vi "Move Robot.vi"(0 "Power (-100 to 100)\n0 = Stop/Brake\n-128 = Stop/Coast":i8(slide) scale=-100.0..100.0, 1 "Mode":enum16{"Constent Speed", "Rotation", "Stop"}(ring), 2 "Move mode":T1(ring), 3 "Robot Target (mm,Rotation)":i32) -> ()   [LabVIEW 2015]
panel:
  out "Busy":bool
  # "1770 = 1 Rotation"
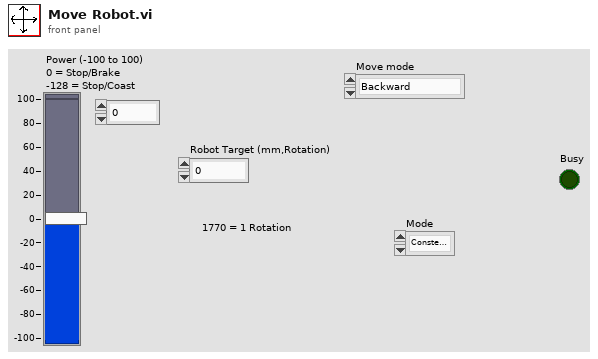
[diagram p1: front panel]
types:
  T1 = enum16{"Backward", "Forward", "Left", "Right", "Rotate Left", "Rotate Right"}
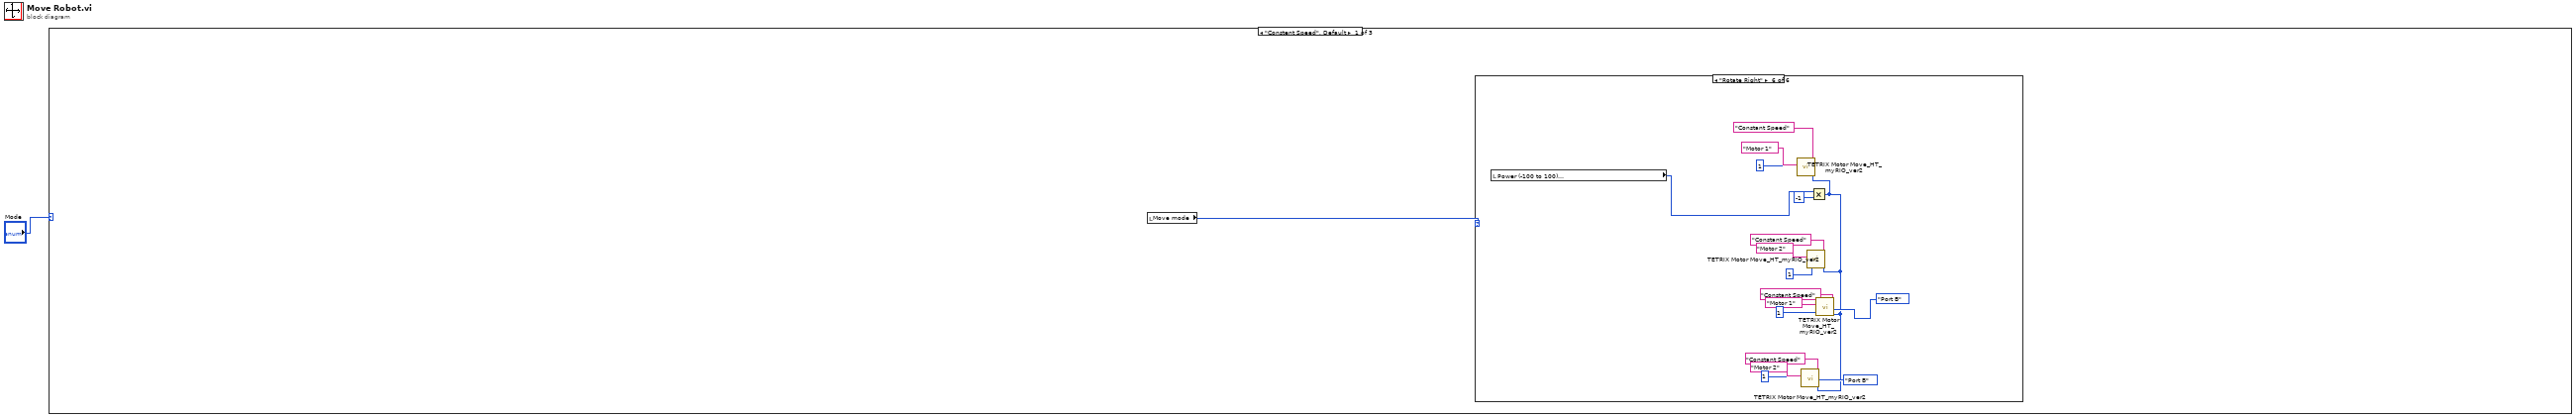
[diagram p0: block diagram]
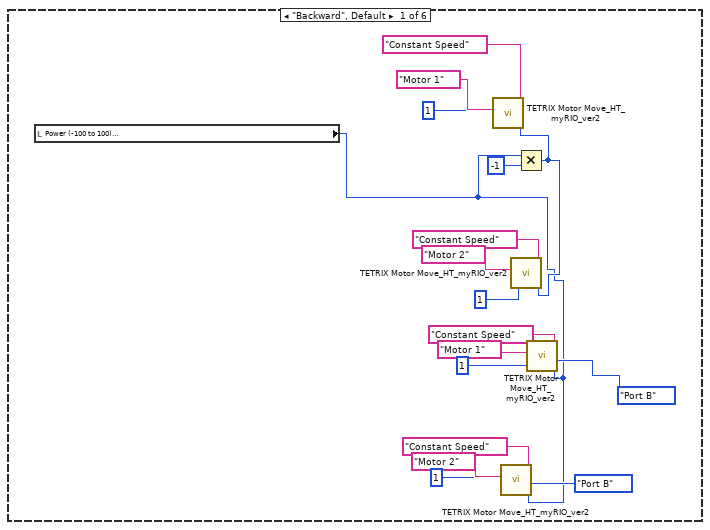
[diagram p2: hidden frame]
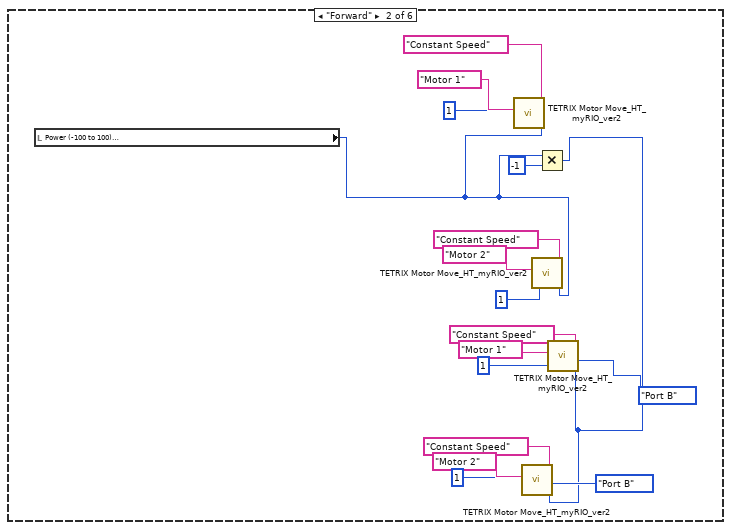
[diagram p3: hidden frame]
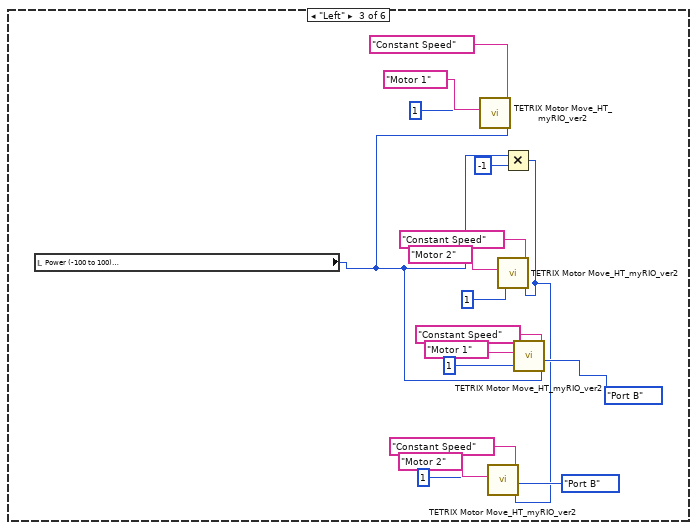
[diagram p4: hidden frame]
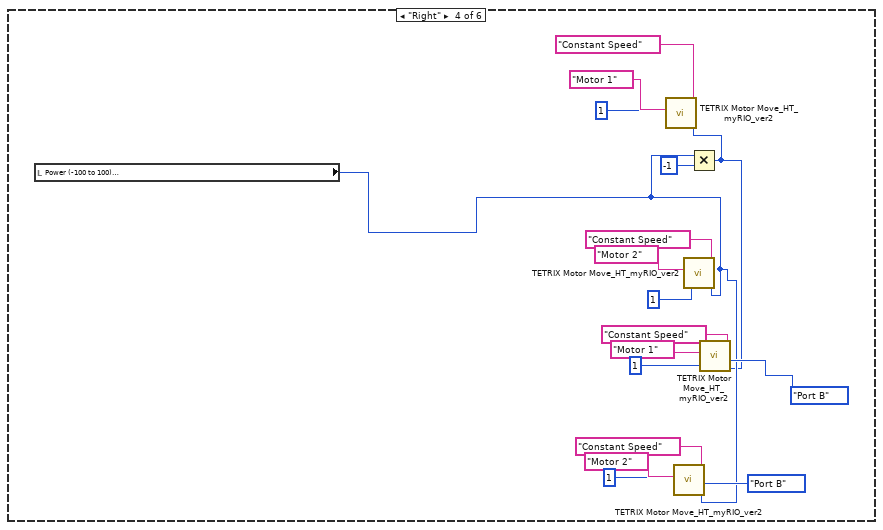
[diagram p5: hidden frame]
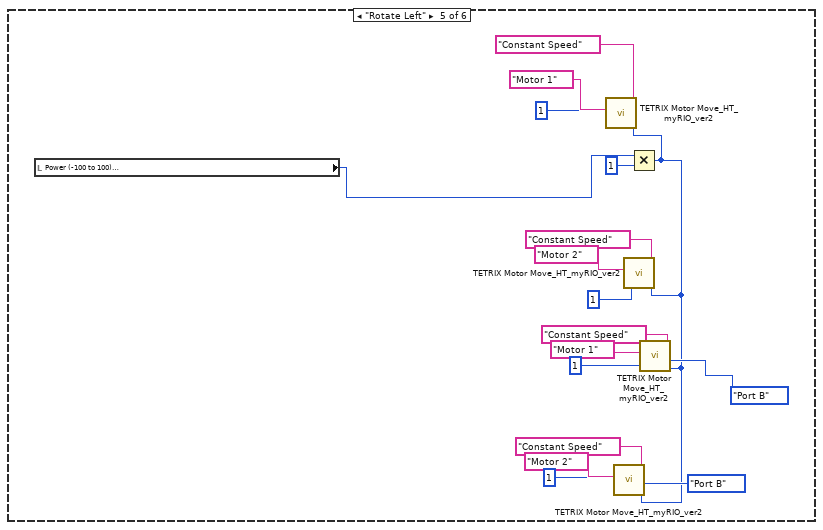
[diagram p6: hidden frame]
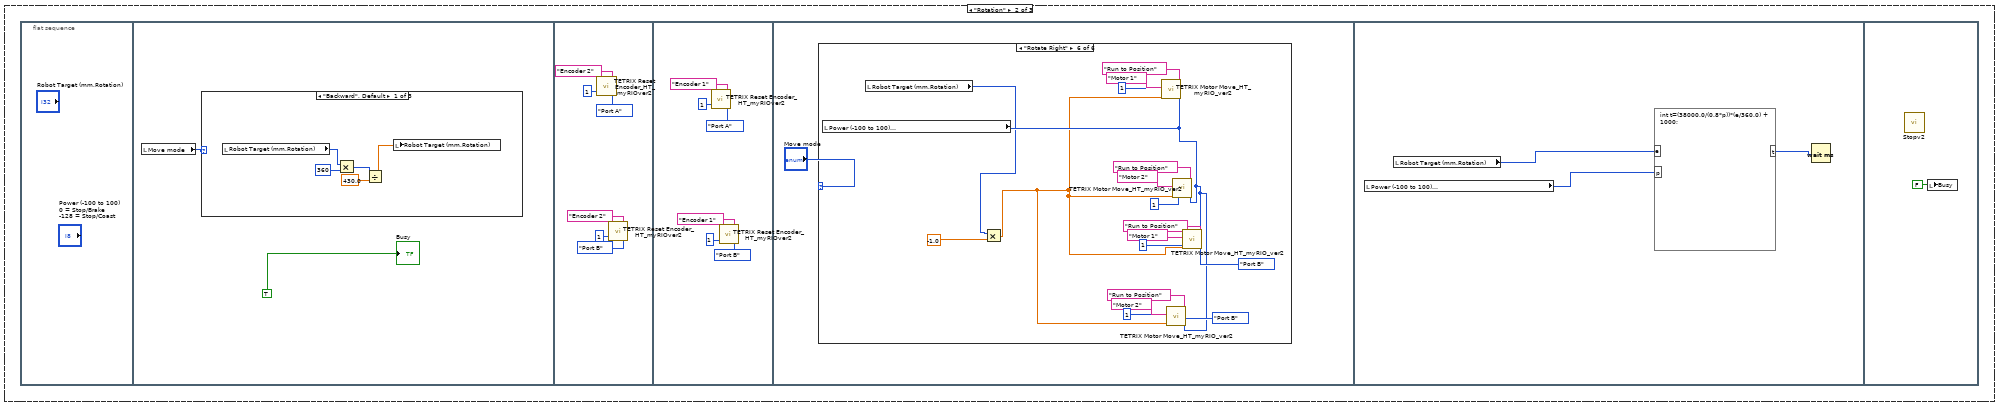
[diagram p7: hidden frame]
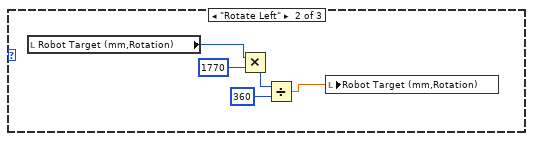
[diagram p8: hidden frame]
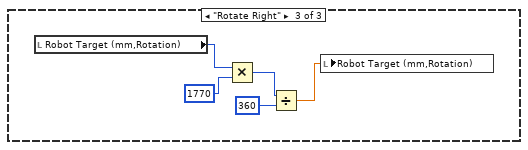
[diagram p9: hidden frame]
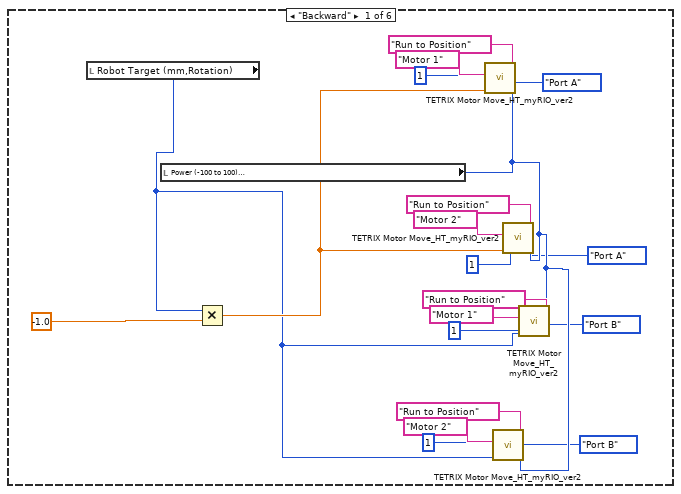
[diagram p10: hidden frame]
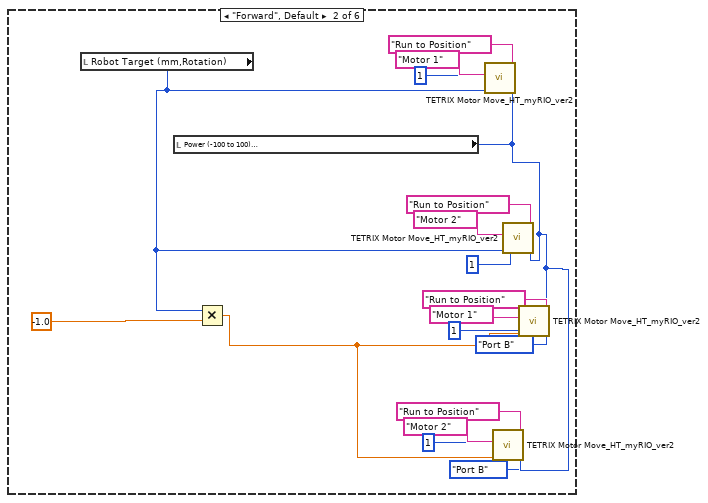
[diagram p11: hidden frame]
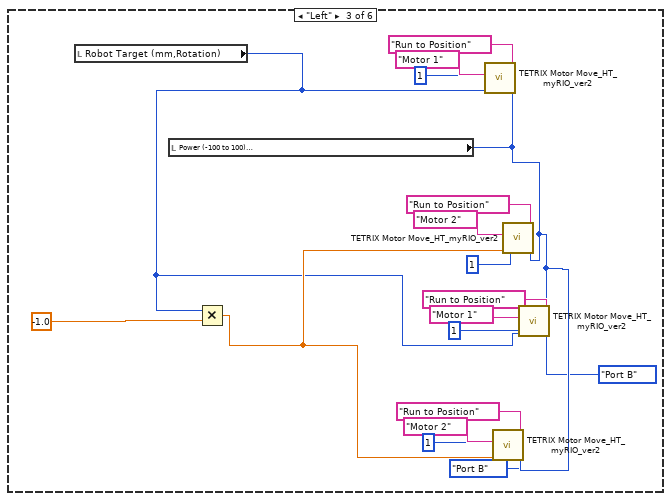
[diagram p12: hidden frame]
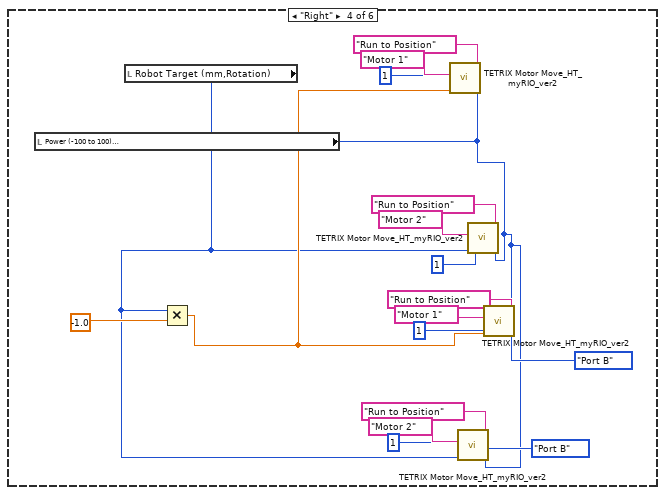
[diagram p13: hidden frame]
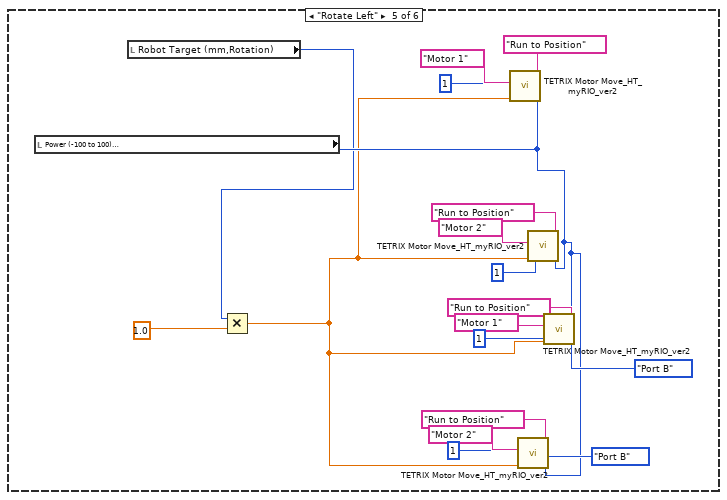
[diagram p14: hidden frame]
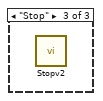
[diagram p15: hidden frame]
diagram:
  n1 = case shown="\"Constent Speed\", Default" "Mode" {
    frame "Constent Speed", Default {
      n2 = local read "Move mode"() -> (w2:T1)
      n3 = case shown="\"Rotate Right\"" w2 {
        frame "Backward", Default {
          n4 = local read "Power (-100 to 100)\n0 = Stop/Brake\n-128 = Stop/Coast"() -> (w3:i8)
          n5 = call "TETRIX Motor Move_HT_myRIO_ver2.vi"("Select Channel"="Motor 2", "Controller Daisy Chain Position: 1 - 4"=u8 1, "Control Mode"="Constant Speed", "Port"=enum16{"Port A", "Port B", ""}."Port B", "Power (-100 to 100)\n0 = Stop/Brake\n-128 = Stop/Coast"=w3) -> ()  [unwired: 3 in, 1 out]
          n6 = Multiply(x=w3, y=i8 -1) -> (x*y=w4:i8)
          n7 = call "TETRIX Motor Move_HT_myRIO_ver2.vi"("Select Channel"="Motor 1", "Controller Daisy Chain Position: 1 - 4"=u8 1, "Control Mode"="Constant Speed", "Power (-100 to 100)\n0 = Stop/Brake\n-128 = Stop/Coast"=w4) -> ()  [unwired: 4 in, 1 out]
          n8 = call "TETRIX Motor Move_HT_myRIO_ver2.vi"("Select Channel"="Motor 2", "Controller Daisy Chain Position: 1 - 4"=u8 1, "Control Mode"="Constant Speed", "Power (-100 to 100)\n0 = Stop/Brake\n-128 = Stop/Coast"=w4) -> ()  [unwired: 4 in, 1 out]
          n9 = call "TETRIX Motor Move_HT_myRIO_ver2.vi"("Select Channel"="Motor 1", "Controller Daisy Chain Position: 1 - 4"=u8 1, "Control Mode"="Constant Speed", "Port"=enum16{"Port A", "Port B", ""}."Port B", "Power (-100 to 100)\n0 = Stop/Brake\n-128 = Stop/Coast"=w3) -> ()  [unwired: 3 in, 1 out]
        }
        frame "Forward" {
          n10 = local read "Power (-100 to 100)\n0 = Stop/Brake\n-128 = Stop/Coast"() -> (w20:i8)
          n11 = call "TETRIX Motor Move_HT_myRIO_ver2.vi"("Select Channel"="Motor 1", "Controller Daisy Chain Position: 1 - 4"=u8 1, "Control Mode"="Constant Speed", "Power (-100 to 100)\n0 = Stop/Brake\n-128 = Stop/Coast"=w20) -> ()  [unwired: 4 in, 1 out]
          n12 = call "TETRIX Motor Move_HT_myRIO_ver2.vi"("Select Channel"="Motor 2", "Controller Daisy Chain Position: 1 - 4"=u8 1, "Control Mode"="Constant Speed", "Power (-100 to 100)\n0 = Stop/Brake\n-128 = Stop/Coast"=w20) -> ()  [unwired: 4 in, 1 out]
          n13 = Multiply(x=w20, y=i8 -1) -> (x*y=w21:i8)
          n14 = call "TETRIX Motor Move_HT_myRIO_ver2.vi"("Select Channel"="Motor 2", "Controller Daisy Chain Position: 1 - 4"=u8 1, "Control Mode"="Constant Speed", "Port"=enum16{"Port A", "Port B", ""}."Port B", "Power (-100 to 100)\n0 = Stop/Brake\n-128 = Stop/Coast"=w21) -> ()  [unwired: 3 in, 1 out]
          n15 = call "TETRIX Motor Move_HT_myRIO_ver2.vi"("Select Channel"="Motor 1", "Controller Daisy Chain Position: 1 - 4"=u8 1, "Control Mode"="Constant Speed", "Port"=enum16{"Port A", "Port B", ""}."Port B", "Power (-100 to 100)\n0 = Stop/Brake\n-128 = Stop/Coast"=w21) -> ()  [unwired: 3 in, 1 out]
        }
        frame "Left" {
          n16 = local read "Power (-100 to 100)\n0 = Stop/Brake\n-128 = Stop/Coast"() -> (w37:i8)
          n17 = call "TETRIX Motor Move_HT_myRIO_ver2.vi"("Select Channel"="Motor 1", "Controller Daisy Chain Position: 1 - 4"=u8 1, "Control Mode"="Constant Speed", "Power (-100 to 100)\n0 = Stop/Brake\n-128 = Stop/Coast"=w37) -> ()  [unwired: 4 in, 1 out]
          n18 = Multiply(x=w37, y=i8 -1) -> (x*y=w38:i8)
          n19 = call "TETRIX Motor Move_HT_myRIO_ver2.vi"("Select Channel"="Motor 2", "Controller Daisy Chain Position: 1 - 4"=u8 1, "Control Mode"="Constant Speed", "Port"=enum16{"Port A", "Port B", ""}."Port B", "Power (-100 to 100)\n0 = Stop/Brake\n-128 = Stop/Coast"=w38) -> ()  [unwired: 3 in, 1 out]
          n20 = call "TETRIX Motor Move_HT_myRIO_ver2.vi"("Select Channel"="Motor 2", "Controller Daisy Chain Position: 1 - 4"=u8 1, "Control Mode"="Constant Speed", "Power (-100 to 100)\n0 = Stop/Brake\n-128 = Stop/Coast"=w38) -> ()  [unwired: 4 in, 1 out]
          n21 = call "TETRIX Motor Move_HT_myRIO_ver2.vi"("Select Channel"="Motor 1", "Controller Daisy Chain Position: 1 - 4"=u8 1, "Control Mode"="Constant Speed", "Port"=enum16{"Port A", "Port B", ""}."Port B", "Power (-100 to 100)\n0 = Stop/Brake\n-128 = Stop/Coast"=w37) -> ()  [unwired: 3 in, 1 out]
        }
        frame "Right" {
          n22 = local read "Power (-100 to 100)\n0 = Stop/Brake\n-128 = Stop/Coast"() -> (w56:i8)
          n23 = call "TETRIX Motor Move_HT_myRIO_ver2.vi"("Select Channel"="Motor 2", "Controller Daisy Chain Position: 1 - 4"=u8 1, "Control Mode"="Constant Speed", "Port"=enum16{"Port A", "Port B", ""}."Port B", "Power (-100 to 100)\n0 = Stop/Brake\n-128 = Stop/Coast"=w56) -> ()  [unwired: 3 in, 1 out]
          n24 = call "TETRIX Motor Move_HT_myRIO_ver2.vi"("Select Channel"="Motor 2", "Controller Daisy Chain Position: 1 - 4"=u8 1, "Control Mode"="Constant Speed", "Power (-100 to 100)\n0 = Stop/Brake\n-128 = Stop/Coast"=w56) -> ()  [unwired: 4 in, 1 out]
          n25 = Multiply(x=w56, y=i8 -1) -> (x*y=w54:i8)
          n26 = call "TETRIX Motor Move_HT_myRIO_ver2.vi"("Select Channel"="Motor 1", "Controller Daisy Chain Position: 1 - 4"=u8 1, "Control Mode"="Constant Speed", "Power (-100 to 100)\n0 = Stop/Brake\n-128 = Stop/Coast"=w54) -> ()  [unwired: 4 in, 1 out]
          n27 = call "TETRIX Motor Move_HT_myRIO_ver2.vi"("Select Channel"="Motor 1", "Controller Daisy Chain Position: 1 - 4"=u8 1, "Control Mode"="Constant Speed", "Port"=enum16{"Port A", "Port B", ""}."Port B", "Power (-100 to 100)\n0 = Stop/Brake\n-128 = Stop/Coast"=w54) -> ()  [unwired: 3 in, 1 out]
        }
        frame "Rotate Left" {
          n28 = local read "Power (-100 to 100)\n0 = Stop/Brake\n-128 = Stop/Coast"() -> (w72:i8)
          n29 = Multiply(x=w72, y=i8 1) -> (x*y=w71:i8)
          n30 = call "TETRIX Motor Move_HT_myRIO_ver2.vi"("Select Channel"="Motor 1", "Controller Daisy Chain Position: 1 - 4"=u8 1, "Control Mode"="Constant Speed", "Power (-100 to 100)\n0 = Stop/Brake\n-128 = Stop/Coast"=w71) -> ()  [unwired: 4 in, 1 out]
          n31 = call "TETRIX Motor Move_HT_myRIO_ver2.vi"("Select Channel"="Motor 2", "Controller Daisy Chain Position: 1 - 4"=u8 1, "Control Mode"="Constant Speed", "Port"=enum16{"Port A", "Port B", ""}."Port B", "Power (-100 to 100)\n0 = Stop/Brake\n-128 = Stop/Coast"=w71) -> ()  [unwired: 3 in, 1 out]
          n32 = call "TETRIX Motor Move_HT_myRIO_ver2.vi"("Select Channel"="Motor 2", "Controller Daisy Chain Position: 1 - 4"=u8 1, "Control Mode"="Constant Speed", "Power (-100 to 100)\n0 = Stop/Brake\n-128 = Stop/Coast"=w71) -> ()  [unwired: 4 in, 1 out]
          n33 = call "TETRIX Motor Move_HT_myRIO_ver2.vi"("Select Channel"="Motor 1", "Controller Daisy Chain Position: 1 - 4"=u8 1, "Control Mode"="Constant Speed", "Port"=enum16{"Port A", "Port B", ""}."Port B", "Power (-100 to 100)\n0 = Stop/Brake\n-128 = Stop/Coast"=w71) -> ()  [unwired: 3 in, 1 out]
        }
        frame "Rotate Right" {
          n34 = local read "Power (-100 to 100)\n0 = Stop/Brake\n-128 = Stop/Coast"() -> (w88:i8)
          n35 = Multiply(x=w88, y=i8 -1) -> (x*y=w89:i8)
          n36 = call "TETRIX Motor Move_HT_myRIO_ver2.vi"("Select Channel"="Motor 1", "Controller Daisy Chain Position: 1 - 4"=u8 1, "Control Mode"="Constant Speed", "Power (-100 to 100)\n0 = Stop/Brake\n-128 = Stop/Coast"=w89) -> ()  [unwired: 4 in, 1 out]
          n37 = call "TETRIX Motor Move_HT_myRIO_ver2.vi"("Select Channel"="Motor 2", "Controller Daisy Chain Position: 1 - 4"=u8 1, "Control Mode"="Constant Speed", "Port"=enum16{"Port A", "Port B", ""}."Port B", "Power (-100 to 100)\n0 = Stop/Brake\n-128 = Stop/Coast"=w89) -> ()  [unwired: 3 in, 1 out]
          n38 = call "TETRIX Motor Move_HT_myRIO_ver2.vi"("Select Channel"="Motor 2", "Controller Daisy Chain Position: 1 - 4"=u8 1, "Control Mode"="Constant Speed", "Power (-100 to 100)\n0 = Stop/Brake\n-128 = Stop/Coast"=w89) -> ()  [unwired: 4 in, 1 out]
          n39 = call "TETRIX Motor Move_HT_myRIO_ver2.vi"("Select Channel"="Motor 1", "Controller Daisy Chain Position: 1 - 4"=u8 1, "Control Mode"="Constant Speed", "Port"=enum16{"Port A", "Port B", ""}."Port B", "Power (-100 to 100)\n0 = Stop/Brake\n-128 = Stop/Coast"=w89) -> ()  [unwired: 3 in, 1 out]
        }
      }
    }
    frame "Rotation" {
      n40 = flat-sequence {
        frame #0 {
        }
        frame #1 {
          n41 = local read "Move mode"() -> (w105:T1)
          n42 = case shown="\"Backward\", Default" w105 {
            frame "Backward", Default {
              n43 = local read "Robot Target (mm,Rotation)"() -> (w108:i32)
              n44 = Multiply(x=w108, y=360) -> (x*y=w109:i32)
              n45 = Divide(x=w109, y=430.0) -> (x/y=w107:dbl)
              n46 = local write "Robot Target (mm,Rotation)"(w107) -> ()
            }
            frame "Rotate Left" {
              n47 = local read "Robot Target (mm,Rotation)"() -> (w116:i32)
              n48 = Multiply(x=w116, y=1770) -> (x*y=w114:i32)
              n49 = Divide(x=w114, y=360) -> (x/y=w112:dbl)
              n50 = local write "Robot Target (mm,Rotation)"(w112) -> ()
            }
            frame "Rotate Right" {
              n51 = local read "Robot Target (mm,Rotation)"() -> (w121:i32)
              n52 = Multiply(x=w121, y=1770) -> (x*y=w119:i32)
              n53 = Divide(x=w119, y=360) -> (x/y=w117:dbl)
              n54 = local write "Robot Target (mm,Rotation)"(w117) -> ()
            }
          }
          "Busy" <- TRUE ("Busy")
        }
        frame #2 {
          n55 = call "TETRIX Reset Encoder_HT_myRIOver2.vi"("Controller Daisy Chain Position ( 1 - 4)"=u8 1, "Select Encoder"="Encoder 2", "Port"=enum16{"Port A", "Port B"}."Port A") -> ()  [unwired: 1 in, 1 out]
          n56 = call "TETRIX Reset Encoder_HT_myRIOver2.vi"("Controller Daisy Chain Position ( 1 - 4)"=u8 1, "Select Encoder"="Encoder 2", "Port"=enum16{"Port A", "Port B"}."Port B") -> ()  [unwired: 1 in, 1 out]
        }
        frame #3 {
          n57 = call "TETRIX Reset Encoder_HT_myRIOver2.vi"("Controller Daisy Chain Position ( 1 - 4)"=u8 1, "Select Encoder"="Encoder 1", "Port"=enum16{"Port A", "Port B"}."Port A") -> ()  [unwired: 1 in, 1 out]
          n58 = call "TETRIX Reset Encoder_HT_myRIOver2.vi"("Controller Daisy Chain Position ( 1 - 4)"=u8 1, "Select Encoder"="Encoder 1", "Port"=enum16{"Port A", "Port B"}."Port B") -> ()  [unwired: 1 in, 1 out]
        }
        frame #4 {
          n59 = case shown="\"Rotate Right\"" "Move mode" {
            frame "Backward" {
              n60 = local read "Robot Target (mm,Rotation)"() -> (w135:i32)
              n61 = local read "Power (-100 to 100)\n0 = Stop/Brake\n-128 = Stop/Coast"() -> (w140:i8)
              n62 = Multiply(x=w135, y=-1.0) -> (x*y=w141:dbl)
              n63 = call "TETRIX Motor Move_HT_myRIO_ver2.vi"("Select Channel"="Motor 1", "Controller Daisy Chain Position: 1 - 4"=u8 1, "Encoder Target: 360 = 1 motor shaft revolution"=w141, "Control Mode"="Run to Position", "Port"=enum16{"Port A", "Port B", ""}."Port A", "Power (-100 to 100)\n0 = Stop/Brake\n-128 = Stop/Coast"=w140) -> ()  [unwired: 2 in, 1 out]
              n64 = call "TETRIX Motor Move_HT_myRIO_ver2.vi"("Select Channel"="Motor 2", "Controller Daisy Chain Position: 1 - 4"=u8 1, "Encoder Target: 360 = 1 motor shaft revolution"=w135, "Control Mode"="Run to Position", "Port"=enum16{"Port A", "Port B", ""}."Port B", "Power (-100 to 100)\n0 = Stop/Brake\n-128 = Stop/Coast"=w140) -> ()  [unwired: 2 in, 1 out]
              n65 = call "TETRIX Motor Move_HT_myRIO_ver2.vi"("Select Channel"="Motor 2", "Controller Daisy Chain Position: 1 - 4"=u8 1, "Encoder Target: 360 = 1 motor shaft revolution"=w141, "Control Mode"="Run to Position", "Port"=enum16{"Port A", "Port B", ""}."Port A", "Power (-100 to 100)\n0 = Stop/Brake\n-128 = Stop/Coast"=w140) -> ()  [unwired: 2 in, 1 out]
              n66 = call "TETRIX Motor Move_HT_myRIO_ver2.vi"("Select Channel"="Motor 1", "Controller Daisy Chain Position: 1 - 4"=u8 1, "Encoder Target: 360 = 1 motor shaft revolution"=w135, "Control Mode"="Run to Position", "Port"=enum16{"Port A", "Port B", ""}."Port B", "Power (-100 to 100)\n0 = Stop/Brake\n-128 = Stop/Coast"=w140) -> ()  [unwired: 2 in, 1 out]
            }
            frame "Forward", Default {
              n67 = local read "Robot Target (mm,Rotation)"() -> (w158:i32)
              n68 = local read "Power (-100 to 100)\n0 = Stop/Brake\n-128 = Stop/Coast"() -> (w157:i8)
              n69 = Multiply(x=w158, y=-1.0) -> (x*y=w159:dbl)
              n70 = call "TETRIX Motor Move_HT_myRIO_ver2.vi"("Select Channel"="Motor 1", "Controller Daisy Chain Position: 1 - 4"=u8 1, "Encoder Target: 360 = 1 motor shaft revolution"=w158, "Control Mode"="Run to Position", "Power (-100 to 100)\n0 = Stop/Brake\n-128 = Stop/Coast"=w157) -> ()  [unwired: 3 in, 1 out]
              n71 = call "TETRIX Motor Move_HT_myRIO_ver2.vi"("Select Channel"="Motor 2", "Controller Daisy Chain Position: 1 - 4"=u8 1, "Encoder Target: 360 = 1 motor shaft revolution"=w159, "Control Mode"="Run to Position", "Port"=enum16{"Port A", "Port B", ""}."Port B", "Power (-100 to 100)\n0 = Stop/Brake\n-128 = Stop/Coast"=w157) -> ()  [unwired: 2 in, 1 out]
              n72 = call "TETRIX Motor Move_HT_myRIO_ver2.vi"("Select Channel"="Motor 2", "Controller Daisy Chain Position: 1 - 4"=u8 1, "Encoder Target: 360 = 1 motor shaft revolution"=w158, "Control Mode"="Run to Position", "Power (-100 to 100)\n0 = Stop/Brake\n-128 = Stop/Coast"=w157) -> ()  [unwired: 3 in, 1 out]
              n73 = call "TETRIX Motor Move_HT_myRIO_ver2.vi"("Select Channel"="Motor 1", "Controller Daisy Chain Position: 1 - 4"=u8 1, "Encoder Target: 360 = 1 motor shaft revolution"=w159, "Control Mode"="Run to Position", "Port"=enum16{"Port A", "Port B", ""}."Port B", "Power (-100 to 100)\n0 = Stop/Brake\n-128 = Stop/Coast"=w157) -> ()  [unwired: 2 in, 1 out]
            }
            frame "Left" {
              n74 = local read "Robot Target (mm,Rotation)"() -> (w173:i32)
              n75 = local read "Power (-100 to 100)\n0 = Stop/Brake\n-128 = Stop/Coast"() -> (w176:i8)
              n76 = Multiply(x=w173, y=-1.0) -> (x*y=w177:dbl)
              n77 = call "TETRIX Motor Move_HT_myRIO_ver2.vi"("Select Channel"="Motor 1", "Controller Daisy Chain Position: 1 - 4"=u8 1, "Encoder Target: 360 = 1 motor shaft revolution"=w173, "Control Mode"="Run to Position", "Power (-100 to 100)\n0 = Stop/Brake\n-128 = Stop/Coast"=w176) -> ()  [unwired: 3 in, 1 out]
              n78 = call "TETRIX Motor Move_HT_myRIO_ver2.vi"("Select Channel"="Motor 2", "Controller Daisy Chain Position: 1 - 4"=u8 1, "Encoder Target: 360 = 1 motor shaft revolution"=w177, "Control Mode"="Run to Position", "Port"=enum16{"Port A", "Port B", ""}."Port B", "Power (-100 to 100)\n0 = Stop/Brake\n-128 = Stop/Coast"=w176) -> ()  [unwired: 2 in, 1 out]
              n79 = call "TETRIX Motor Move_HT_myRIO_ver2.vi"("Select Channel"="Motor 2", "Controller Daisy Chain Position: 1 - 4"=u8 1, "Encoder Target: 360 = 1 motor shaft revolution"=w177, "Control Mode"="Run to Position", "Power (-100 to 100)\n0 = Stop/Brake\n-128 = Stop/Coast"=w176) -> ()  [unwired: 3 in, 1 out]
              n80 = call "TETRIX Motor Move_HT_myRIO_ver2.vi"("Select Channel"="Motor 1", "Controller Daisy Chain Position: 1 - 4"=u8 1, "Encoder Target: 360 = 1 motor shaft revolution"=w173, "Control Mode"="Run to Position", "Port"=enum16{"Port A", "Port B", ""}."Port B", "Power (-100 to 100)\n0 = Stop/Brake\n-128 = Stop/Coast"=w176) -> ()  [unwired: 2 in, 1 out]
            }
            frame "Right" {
              n81 = local read "Power (-100 to 100)\n0 = Stop/Brake\n-128 = Stop/Coast"() -> (w192:i8)
              n82 = local read "Robot Target (mm,Rotation)"() -> (w191:i32)
              n83 = Multiply(x=w191, y=-1.0) -> (x*y=w195:dbl)
              n84 = call "TETRIX Motor Move_HT_myRIO_ver2.vi"("Select Channel"="Motor 1", "Controller Daisy Chain Position: 1 - 4"=u8 1, "Encoder Target: 360 = 1 motor shaft revolution"=w195, "Control Mode"="Run to Position", "Power (-100 to 100)\n0 = Stop/Brake\n-128 = Stop/Coast"=w192) -> ()  [unwired: 3 in, 1 out]
              n85 = call "TETRIX Motor Move_HT_myRIO_ver2.vi"("Select Channel"="Motor 2", "Controller Daisy Chain Position: 1 - 4"=u8 1, "Encoder Target: 360 = 1 motor shaft revolution"=w191, "Control Mode"="Run to Position", "Port"=enum16{"Port A", "Port B", ""}."Port B", "Power (-100 to 100)\n0 = Stop/Brake\n-128 = Stop/Coast"=w192) -> ()  [unwired: 2 in, 1 out]
              n86 = call "TETRIX Motor Move_HT_myRIO_ver2.vi"("Select Channel"="Motor 2", "Controller Daisy Chain Position: 1 - 4"=u8 1, "Encoder Target: 360 = 1 motor shaft revolution"=w191, "Control Mode"="Run to Position", "Power (-100 to 100)\n0 = Stop/Brake\n-128 = Stop/Coast"=w192) -> ()  [unwired: 3 in, 1 out]
              n87 = call "TETRIX Motor Move_HT_myRIO_ver2.vi"("Select Channel"="Motor 1", "Controller Daisy Chain Position: 1 - 4"=u8 1, "Encoder Target: 360 = 1 motor shaft revolution"=w195, "Control Mode"="Run to Position", "Port"=enum16{"Port A", "Port B", ""}."Port B", "Power (-100 to 100)\n0 = Stop/Brake\n-128 = Stop/Coast"=w192) -> ()  [unwired: 2 in, 1 out]
            }
            frame "Rotate Left" {
              n88 = local read "Power (-100 to 100)\n0 = Stop/Brake\n-128 = Stop/Coast"() -> (w211:i8)
              n89 = local read "Robot Target (mm,Rotation)"() -> (w209:i32)
              n90 = Multiply(x=w209, y=1.0) -> (x*y=w210:dbl)
              n91 = call "TETRIX Motor Move_HT_myRIO_ver2.vi"("Select Channel"="Motor 1", "Controller Daisy Chain Position: 1 - 4"=u8 1, "Encoder Target: 360 = 1 motor shaft revolution"=w210, "Control Mode"="Run to Position", "Power (-100 to 100)\n0 = Stop/Brake\n-128 = Stop/Coast"=w211) -> ()  [unwired: 3 in, 1 out]
              n92 = call "TETRIX Motor Move_HT_myRIO_ver2.vi"("Select Channel"="Motor 2", "Controller Daisy Chain Position: 1 - 4"=u8 1, "Encoder Target: 360 = 1 motor shaft revolution"=w210, "Control Mode"="Run to Position", "Port"=enum16{"Port A", "Port B", ""}."Port B", "Power (-100 to 100)\n0 = Stop/Brake\n-128 = Stop/Coast"=w211) -> ()  [unwired: 2 in, 1 out]
              n93 = call "TETRIX Motor Move_HT_myRIO_ver2.vi"("Select Channel"="Motor 2", "Controller Daisy Chain Position: 1 - 4"=u8 1, "Encoder Target: 360 = 1 motor shaft revolution"=w210, "Control Mode"="Run to Position", "Power (-100 to 100)\n0 = Stop/Brake\n-128 = Stop/Coast"=w211) -> ()  [unwired: 3 in, 1 out]
              n94 = call "TETRIX Motor Move_HT_myRIO_ver2.vi"("Select Channel"="Motor 1", "Controller Daisy Chain Position: 1 - 4"=u8 1, "Encoder Target: 360 = 1 motor shaft revolution"=w210, "Control Mode"="Run to Position", "Port"=enum16{"Port A", "Port B", ""}."Port B", "Power (-100 to 100)\n0 = Stop/Brake\n-128 = Stop/Coast"=w211) -> ()  [unwired: 2 in, 1 out]
            }
            frame "Rotate Right" {
              n95 = local read "Power (-100 to 100)\n0 = Stop/Brake\n-128 = Stop/Coast"() -> (w229:i8)
              n96 = local read "Robot Target (mm,Rotation)"() -> (w227:i32)
              n97 = Multiply(x=w227, y=-1.0) -> (x*y=w228:dbl)
              n98 = call "TETRIX Motor Move_HT_myRIO_ver2.vi"("Select Channel"="Motor 1", "Controller Daisy Chain Position: 1 - 4"=u8 1, "Encoder Target: 360 = 1 motor shaft revolution"=w228, "Control Mode"="Run to Position", "Power (-100 to 100)\n0 = Stop/Brake\n-128 = Stop/Coast"=w229) -> ()  [unwired: 3 in, 1 out]
              n99 = call "TETRIX Motor Move_HT_myRIO_ver2.vi"("Select Channel"="Motor 2", "Controller Daisy Chain Position: 1 - 4"=u8 1, "Encoder Target: 360 = 1 motor shaft revolution"=w228, "Control Mode"="Run to Position", "Port"=enum16{"Port A", "Port B", ""}."Port B", "Power (-100 to 100)\n0 = Stop/Brake\n-128 = Stop/Coast"=w229) -> ()  [unwired: 2 in, 1 out]
              n100 = call "TETRIX Motor Move_HT_myRIO_ver2.vi"("Select Channel"="Motor 2", "Controller Daisy Chain Position: 1 - 4"=u8 1, "Encoder Target: 360 = 1 motor shaft revolution"=w228, "Control Mode"="Run to Position", "Power (-100 to 100)\n0 = Stop/Brake\n-128 = Stop/Coast"=w229) -> ()  [unwired: 3 in, 1 out]
              n101 = call "TETRIX Motor Move_HT_myRIO_ver2.vi"("Select Channel"="Motor 1", "Controller Daisy Chain Position: 1 - 4"=u8 1, "Encoder Target: 360 = 1 motor shaft revolution"=w228, "Control Mode"="Run to Position", "Port"=enum16{"Port A", "Port B", ""}."Port B", "Power (-100 to 100)\n0 = Stop/Brake\n-128 = Stop/Coast"=w229) -> ()  [unwired: 2 in, 1 out]
            }
          }
        }
        frame #5 {
          n102 = local read "Power (-100 to 100)\n0 = Stop/Brake\n-128 = Stop/Coast"() -> (w246:i8)
          n103 = local read "Robot Target (mm,Rotation)"() -> (w245:i32)
          n104 = formula code="int t=(38000.0/(0.8*p))*(e/360.0) + 1000;"("e"=w245, "p"=w246) -> ("t"=w247:i32)
          n105 = Wait (ms)(milliseconds to wait=w247) -> ()  [unwired: 1 out]
        }
        frame #6 {
          n106 = call "Stopv2.vi"() -> ()  [unwired: 12 in]
          n107 = local write "Busy"(FALSE ("Busy")) -> ()
        }
      }
    }
    frame "Stop" {
      n108 = call "Stopv2.vi"() -> ()  [unwired: 12 in]
    }
  }
